vi "AIS Shielding Box Management.vi"() -> ()   [LabVIEW 2020]
uses:
  Commun VI/TypeDef/Commande Popup autotest/Commande element autotest.ctl
  01 - Structure de base/Fonction/Shielding Box/Action.ctl
  01 - Structure de base/Commande special/Exit.ctl
  01 - Structure de base/IHM/Variable globale.vi
panel:
  out "Element autotest":T1
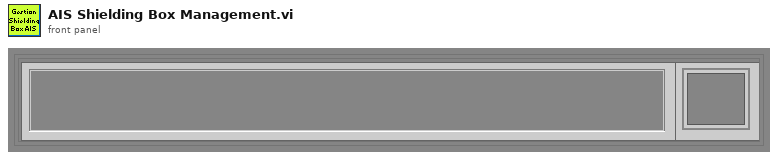
[diagram p1: front panel]
types:
  T1 = typedef "Commande element autotest.ctl" = cluster{"Instrument":string, "Etat":cluster{"Menu déroulant":u16}}
  T2 = typedef "Action.ctl" = enum16{"Open Shielding", "Close Shielding", "Read Status", "Stop Wait Start", "Wait Start", "Wait Close", "Wait Open", "Quit"}
  T3 = typedef "File et notification.ctl" = cluster{"Arret Appli":refnum<notifier>, "Erreur Acqui":refnum<notifier>, "File Event Sequenceur":refnum<queue>, "Liste test à faire":refnum<queue>, "File Event Historique":refnum<queue>, "Variable Global":refnum<notifier>, "Variable stocke retour Etat":refnum<notifier>, "Retour Validation OP":refnum<queue>, "Demande Validation OP":refnum<queue>, "Retour Autotest":refnum<notifier>, "Demande Autotest":refnum<queue>, "Adr Mac Produit":refnum<notifier>, "Autorise commande":refnum<notifier>, "Event Init BLE":refnum<notifier>, "Action Lecture RS":refnum<queue>, "Key produit":refnum<notifier>, "Retour Saisie OP":refnum<queue>, "Demande Saisie OP":refnum<queue>, "Etat flashage":refnum<notifier>, "Code Operateur":refnum<notifier>, "Resultat test Global":refnum<notifier>, "Stop Test":refnum<notifier>, "Init IHM Autotest":refnum<notifier>, "Version test bench":refnum<notifier>, "SN Product":refnum<notifier>, "En erreur":refnum<notifier>, "Affiche Result":refnum<queue>, "S/N PWR":refnum<notifier>, "AppEUI":refnum<notifier>, "Action Lecture Temp":refnum<queue>, "Temp":refnum<notifier>, "AppKey":refnum<notifier>, "OF":refnum<notifier>, "File Commande Shielding":refnum<queue>, "Return Status":refnum<notifier>, "ID Product":refnum<notifier>, "Version FW":refnum<notifier>, "Version HW":refnum<notifier>, "Adresse IHM":refnum<notifier>, "RTC":refnum<notifier>, "S/N Ant":refnum<notifier>, "SN Encode":refnum<notifier>, "Key Product":refnum<notifier>}
  T4 = typedef "Commande Variable Global.ctl" = cluster{"Fichier":cluster{"Chemin Save Historique":path, "Fichier Appplication":string, "Fichier Test":string, "Fichier Langue":string, "Part Number":string, "Fichier Parametre":string, "Chemin Fichier Parametre":path, "Fichier Print":string, "Fichier BDD":string}, "Liaison Serie":cluster{"RS Alimentation":refnum<visa-resource-name>, "RS Multimetre":refnum<k15>, "RS Carte":refnum<visa-resource-name>, "RS Dongle WIFI":refnum<visa-resource-name>, "RS Dongle BLE":refnum<visa-resource-name>, "RSA306":refnum<visa-resource-name>, "RS Printer PCBA":refnum<visa-resource-name>, "RS Golden Sample":refnum<visa-resource-name>, "RS Printer Ass":refnum<visa-resource-name>, "RS Printer Pack":refnum<visa-resource-name>, "RS Sonde Temp":refnum<visa-resource-name>, "RS Multimetre Bis":refnum<k15>, "RS FEASA LED":refnum<visa-resource-name>}, "Liaison DIO":cluster{"Jlink":cluster{"Line":tag, "Nom Voie":string, "Nom device in INI":string}[], "ICD":cluster{"Line":tag, "Nom Voie":string, "Nom device in INI":string}[], "UART":cluster{"Line":tag, "Nom Voie":string, "Nom device in INI":string}[], "Multi1":cluster{"Line":tag, "Nom Voie":string, "Nom device in INI":string}[], "Multi2":cluster{"Line":tag, "Nom Voie":string, "Nom device in INI":string}[], "Multi3":cluster{"Line":tag, "Nom Voie":string, "Nom device in INI":string}[], "DO1":cluster{"Line":tag, "Nom Voie":string, "Nom device in INI":string}[], "DO2":cluster{"Line":tag, "Nom Voie":string, "Nom device in INI":string}[], "DO3":cluster{"Line":tag, "Nom Voie":string, "Nom device in INI":string}[], "AlimProduct":cluster{"Line":tag, "Nom Voie":string, "Nom device in INI":string}[], "SW2":cluster{"Line":tag, "Nom Voie":string, "Nom device in INI":string}[], "SW1":cluster{"Line":tag, "Nom Voie":string, "Nom device in INI":string}[], "Multi220V_CPT":cluster{"Line":tag, "Nom Voie":string, "Nom device in INI":string}[]}, "Variable Programme":T5, "Information Entete":cluster{"Opérateur":string, "Ordre de fabrication":string, "Numéro de lot":string, "Commentaire":string}, "Nom de périphérique DAQmx":tag, "Parameter RF":cluster{"Frequency CW":string, "FrequencyRX":string, "TimeOutRX":string}, "Divers":cluster{"DUT Hub":u32}, "Analogique":cluster{"AI1":cluster{"Voie":tag, "Nom Voie":string, "Nom device in INI":string}[], "Ai2":cluster{"Voie":tag, "Nom Voie":string, "Nom device in INI":string}[], "AI3":cluster{"Voie":tag, "Nom Voie":string, "Nom device in INI":string}[], "AI4":cluster{"Voie":tag, "Nom Voie":string, "Nom device in INI":string}[], "AI5":cluster{"Voie":tag, "Nom Voie":string, "Nom device in INI":string}[], "AI6":cluster{"Voie":tag, "Nom Voie":string, "Nom device in INI":string}[], "AI7":cluster{"Voie":tag, "Nom Voie":string, "Nom device in INI":string}[], "AI8":cluster{"Voie":tag, "Nom Voie":string, "Nom device in INI":string}[], "AO1":cluster{"Voie":tag, "Nom Voie":string, "Nom device in INI":string}[], "AO2":cluster{"Voie":tag, "Nom Voie":string, "Nom device in INI":string}[]}, "Parametre BLE":T8, "Shielding Box":cluster{"Comm":refnum<visa-resource-name>, "Used":bool}, "Challenge Bit":u8[]}
  T5 = typedef "Commande Variables Programme.ctl" = cluster{"Cigarette en cours":i32, "Tableau Resultat test":T6, "Test en cours":i32, "Type test":string, "Type Carte":T7, "Test Select":cluster{"Booléen 4":bool}[]}
  T6 = typedef "Commande tableau Resultat.ctl" = cluster{"Resultat produit":cluster{"Nom test":string, "Result test":bool[], "Nom pointe de test":string[], "Valeur test":string[], "Temps Etape":dbl, "Numero Etape":string[]}[]}[]
  T7 = typedef "Commande Selection produit en cours.ctl" = enum16{"None", "PCBA", "Assembled"}
  T8 = typedef "Comande Variable Globale BLE.ctl" = cluster{"Devices Connect":string[][], "Connection Status":T9, "Handle table":string[][], "Service":string, "characteristic Read":string, "characteristic Write":string, "Port BLE":refnum<visa-resource-name>, "Nb Packet Light":u8}
  T9 = typedef "connection_status_bundle.ctl" = cluster{"MAC Address":string, "cnx handle":u8, "cnx flags":u8, "Address Type":T10, "Connection Interval (ms)":u16, "Timeout(ms)":u16, "Latency":u16, "bonding handle":u8}
  T10 = typedef "address_type.ctl" = u8
  T11 = typedef "Exit.ctl" = bool
  T12 = enum32{"Invalid", "Standard", "Closed", "Hidden", "Minimized", "Maximized"}
  T13 = typedef "Adresse IHM.ctl" = cluster{"TabGestionScénario":refnum<vi>, "MAJ TabTest":refnum<vi>, "MAJ IHM":refnum<vi>, "BpStop":refnum<vi>, "Autotest OK":refnum<vi>, "BpContinue":refnum<vi>, "BpStart":refnum<vi>, "Action en chinois":refnum<vi>, "Bouton vide":refnum<vi>, "StatusPCB":refnum<vi>, "StatusAssembled":refnum<vi>, "Bouton Exit":refnum<vi>, "Action En cours":refnum<vi>}
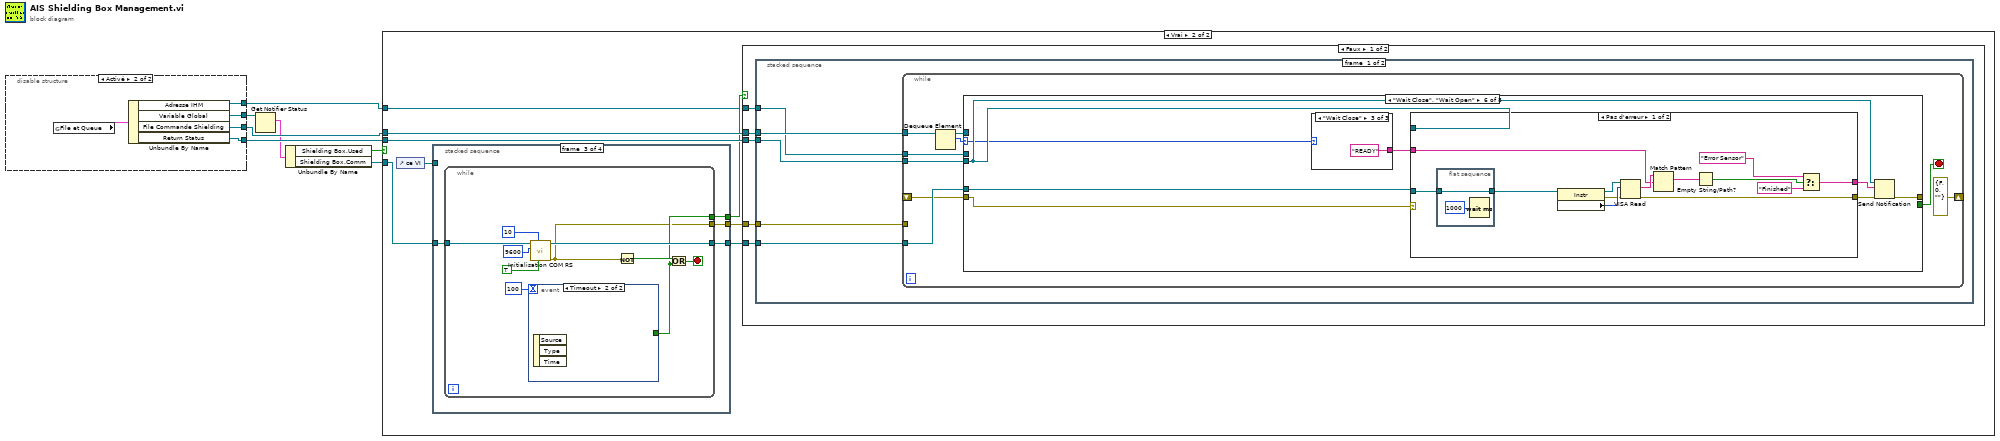
[diagram p0: block diagram]
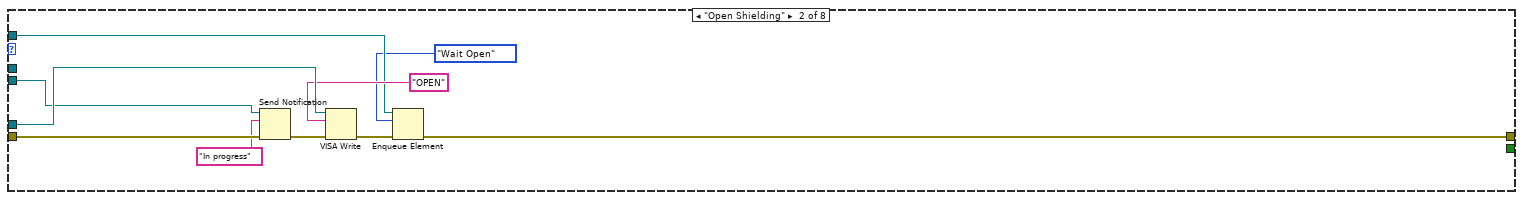
[diagram p4: hidden frame]
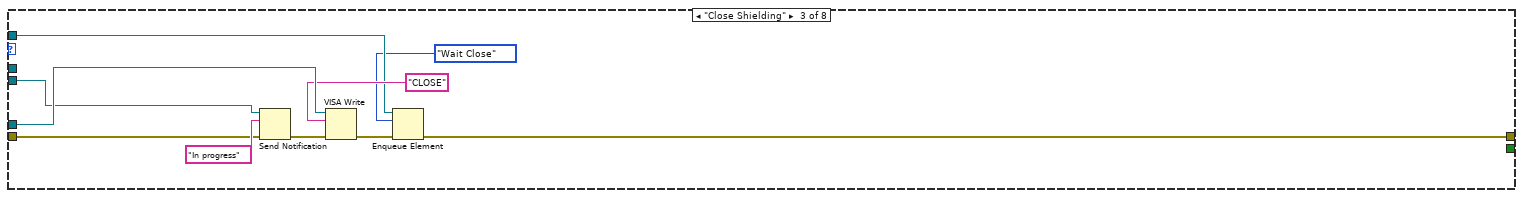
[diagram p5: hidden frame]
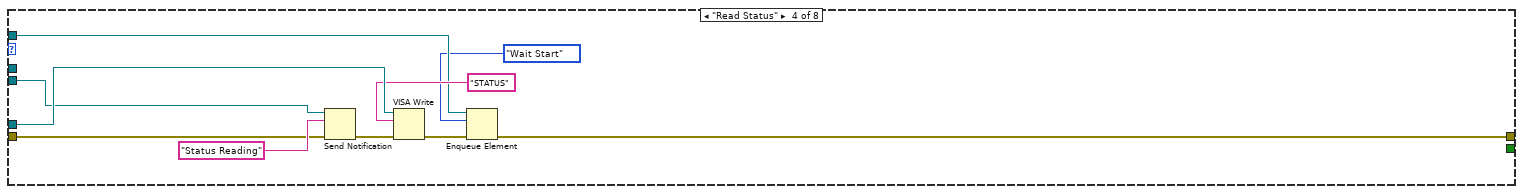
[diagram p6: hidden frame]
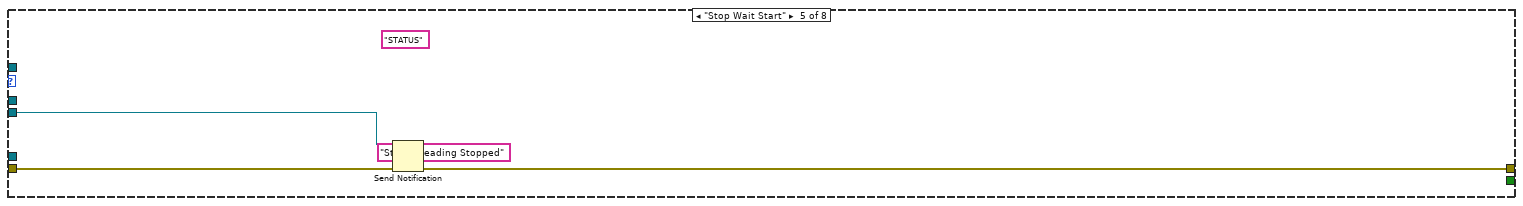
[diagram p7: hidden frame]
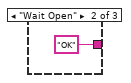
[diagram p9: hidden frame]
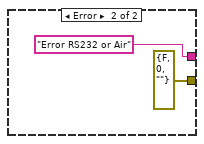
[diagram p10: hidden frame]
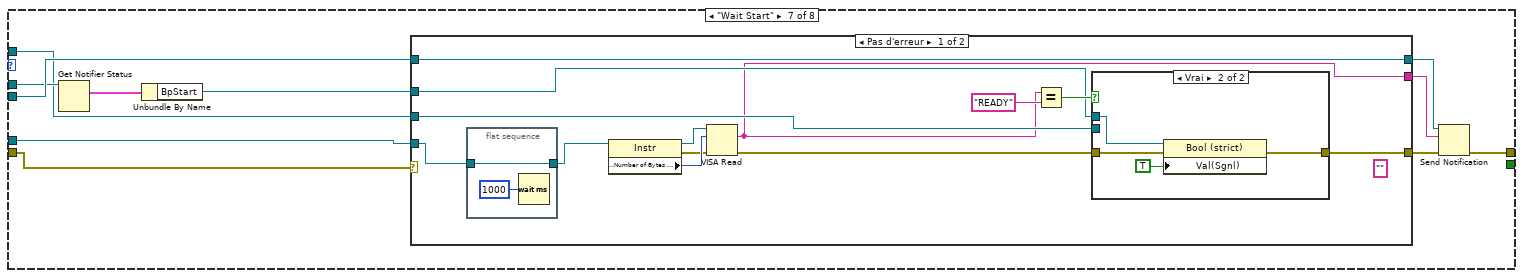
[diagram p11: hidden frame]
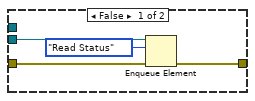
[diagram p12: hidden frame]
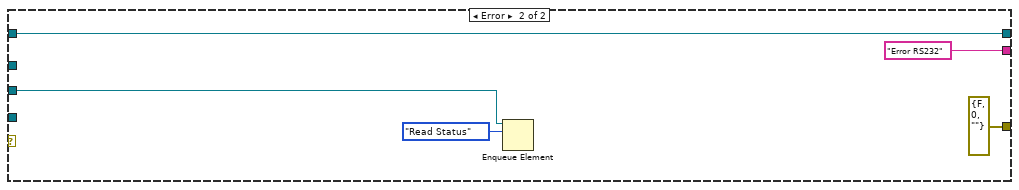
[diagram p13: hidden frame]
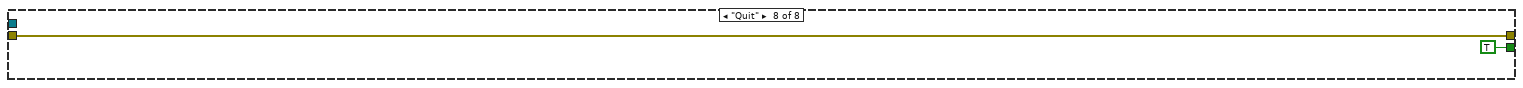
[diagram p14: hidden frame]
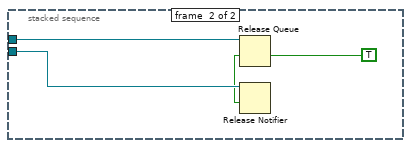
[diagram p15: hidden frame]
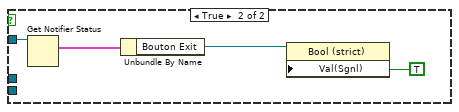
[diagram p16: hidden frame]
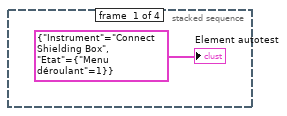
[diagram p17: hidden frame]
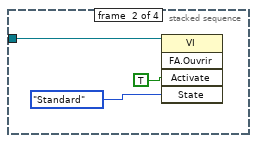
[diagram p18: hidden frame]
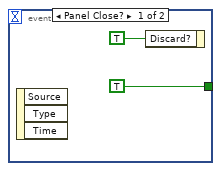
[diagram p19: hidden frame]
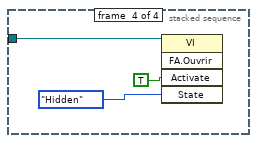
[diagram p20: hidden frame]
diagram:
  n1 = disable-structure shown="Activé" {
    disable-tunnel: [w12 w17] -> w7
    disable-tunnel: [w9 w16] -> w6
    disable-tunnel: [_ w15] -> w5
    disable-tunnel: [_ w14] -> w1
    frame Disabled {
      n2 = Obtain Queue(name (unnamed)="File Commande Shielding" ("nom (aucun)"), element data type=Action."Wait Start") -> (queue out=w12:refnum<queue>)  [unwired: 3 in, 2 out]
      n3 = Obtain Notifier(name (unnamed)="Return Status" ("nom (aucun)"), notification data type="") -> (notifier out=w9:refnum<notifier>)  [unwired: 2 in, 2 out]
    }
    frame Enabled {
      n4 = global read "Variable globale.vi" "File et Queue"() -> (w18:T3)
      n5 = Unbundle By Name(w18) -> ("Adresse IHM"=w14:refnum<notifier>, "Variable Global"=w15:refnum<notifier>, "File Commande Shielding"=w17:refnum<queue>, "Return Status"=w16:refnum<notifier>)
    }
  }
  n6 = Get Notifier Status(notifier=w5) -> (current notification=w3:T4)  [unwired: 1 in, 4 out]
  n7 = Unbundle By Name(w3) -> ("Shielding Box.Used"=w2:bool, "Shielding Box.Comm"=w4:refnum<visa-resource-name>)
  n8 = case shown="Vrai" w2 {
    tunnel: w7 -> [_ w26]
    tunnel: w6 -> [_ w25]
    tunnel: w1 -> [_ w20]
    tunnel: w4 -> [_ w19]
    frame False {
    }
    frame True {
      n9 = control-ref of="ce VI"() -> (w24:refnum<vi>)
      n10 = stacked-sequence {
        tunnel: w24 -> [_ w157 _ w176]
        tunnel: [_ _ w163 _] -> w23
        tunnel: [_ _ w162 _] -> w22
        tunnel: [_ _ w161 _] -> w21
        tunnel: w19 -> [_ _ w160 _]
        frame #0 {
          "Element autotest" <- T1 {"Instrument"="Connect Shielding Box", "Etat"={"Menu déroulant"=1}} ("Element autotest")
        }
        frame #1 {
          n11 = invoke class="VI" method="FA.Ouvrir"(reference=w157, "Activate"=TRUE ("Activer ?"), "State"=T12."Standard" ("État")) -> ()  [unwired: 2 in, 5 out]
        }
        frame #2 {
          n12 = while {
            tunnel: [w164] -> w163
            tunnel: [w170] -> w162
            tunnel: [w167] -> w161
            tunnel: w160 -> [w165]
            stop <- w169 stop-if-true
            n13 = event shown="[1] Timeout" {
              selector: _ -> [_ _]
              dyn-events: _ -> [_ _]
              timeout: 100 -> [_ _]
              tunnel: [TRUE _] -> w167
              event Panel Close? {
                n14 = event-data() -> ()  [unwired: 1 in, 3 out]
                n15 = event-data("Discard?"=TRUE ("Rejeter ?")) -> ()  [unwired: 1 in, 1 out]
              }
              event Timeout {
                n16 = event-data() -> ()  [unwired: 1 in, 3 out]
              }
            }
            n17 = call "Initialisation COM RS.vi"("Enable Termination\nChar (T)"=TRUE ("Enable Termination\nChar (T)"), "termination char\n(0xA = '\\n' = LF)"=u8 10 ("termination char\n(0xA = '\\n' = LF)"), "baud rate (9600)"=9600, "Refnum VISA en entrée"=w165) -> ("sortie d'erreur"=w164:errorcluster, "Nom de ressource VISA en sortie"=w170:refnum<visa-resource-name>)  [unwired: 6 in]
            n18 = Not(x=w164) -> (.not. x?=w168:bool)
            n19 = Or(x=w168, y=w167) -> (x .or. y?=w169:bool)
          }
        }
        frame #3 {
          n20 = invoke class="VI" method="FA.Ouvrir"(reference=w176, "Activate"=TRUE ("Activer ?"), "State"=T12."Hidden" ("État")) -> ()  [unwired: 2 in, 5 out]
        }
      }
      n21 = case shown="Faux" w21 {
        tunnel: w26 -> [w31 _]
        tunnel: w25 -> [w30 _]
        tunnel: w23 -> [w29 _]
        tunnel: w22 -> [w28 _]
        tunnel: w20 -> [w27 w155]
        frame False {
          n22 = stacked-sequence {
            tunnel: w28 -> [w36 _]
            tunnel: w31 -> [w35 w151]
            tunnel: w29 -> [w34 _]
            tunnel: w30 -> [w33 w150]
            tunnel: w27 -> [w32 _]
            frame #0 {
              n23 = while {
                tunnel: w36 -> [w43]
                tunnel: w35 -> [w45]
                shift-right: [errorcluster {"status"=FALSE, "code"=0, "source"=""} ("error out")] -> _
                shift-left: _ -> [w42]
                tunnel: w34 -> [_]
                tunnel: w33 -> [w39]
                tunnel: w32 -> [w37]
                stop <- w40 stop-if-true
                n24 = Dequeue Element(queue=w45) -> (queue out=w41:refnum<queue>, element=w44:T2)  [unwired: 2 in, 2 out]
                n25 = case shown="\"Wait Close\", \"Wait Open\"" w44 {
                  selector: w44 -> [_ _ _ _ _ w86 _ _]
                  tunnel: w43 -> [_ w56 w66 w76 _ w88 w118 _]
                  tunnel: w42 -> [w46 w54 w58 w68 w78 w81 w108 w148]
                  tunnel: [w46 w52 w63 w73 w77 w82 w114 w148] -> _
                  tunnel: w41 -> [_ w51 w62 w72 _ _ w110 _]
                  tunnel: [_ _ _ _ _ _ _ TRUE] -> w40
                  tunnel: w39 -> [_ w48 w59 w69 w79 w87 w117 _]
                  tunnel: w37 -> [_ _ _ _ _ _ w115 _]
                  frame Default {
                  }
                  frame "Open Shielding" {
                    n26 = Send Notification(notification="In progress", notifier=w48, error in (no error)=w54) -> (error out=w49:errorcluster)  [unwired: 1 out]
                    n27 = VISA Write(VISA resource name=w56, write buffer="OPEN" ("buffer d'écriture"), error in (no error)=w49) -> (error out=w53:errorcluster)  [unwired: 2 out]
                    n28 = Enqueue Element(queue=w51, element=Action."Wait Open" ("élément"), error in (no error)=w53) -> (error out=w52:errorcluster)  [unwired: 1 in, 2 out]
                  }
                  frame "Close Shielding" {
                    n29 = Send Notification(notification="In progress", notifier=w59, error in (no error)=w58) -> (error out=w57:errorcluster)  [unwired: 1 out]
                    n30 = VISA Write(VISA resource name=w66, write buffer="CLOSE" ("buffer d'écriture"), error in (no error)=w57) -> (error out=w64:errorcluster)  [unwired: 2 out]
                    n31 = Enqueue Element(queue=w62, element=Action."Wait Close" ("élément"), error in (no error)=w64) -> (error out=w63:errorcluster)  [unwired: 1 in, 2 out]
                  }
                  frame "Read Status" {
                    n32 = Send Notification(notification="Status Reading", notifier=w69, error in (no error)=w68) -> (error out=w67:errorcluster)  [unwired: 1 out]
                    n33 = VISA Write(VISA resource name=w76, write buffer="STATUS" ("buffer d'écriture"), error in (no error)=w67) -> (error out=w74:errorcluster)  [unwired: 2 out]
                    n34 = Enqueue Element(queue=w72, element=Action."Wait Start" ("élément"), error in (no error)=w74) -> (error out=w73:errorcluster)  [unwired: 1 in, 2 out]
                  }
                  frame "Stop Wait Start" {
                    (unwired) "STATUS" ("buffer d'écriture")
                    n35 = Send Notification(notification="Status Reading Stopped", notifier=w79, error in (no error)=w78) -> (error out=w77:errorcluster)  [unwired: 1 out]
                  }
                  frame "Wait Close", "Wait Open" {
                    n36 = case shown="\"Wait Close\"" w86 {
                      tunnel: [_ "OK" ("expression régulière") "READY" ("expression régulière")] -> w85
                      frame Default {
                      }
                      frame "Wait Open" {
                      }
                      frame "Wait Close" {
                      }
                    }
                    n37 = case shown="Pas d'erreur" w81 {
                      tunnel: w88 -> [w92 _]
                      tunnel: w87 -> [_ _]
                      tunnel: w85 -> [w95 _]
                      tunnel: [w94 "Error RS232 or Air" ("cas faux")] -> w84
                      tunnel: [w93 errorcluster {"status"=FALSE, "code"=0, "source"=""} ("error out")] -> w83
                      frame No Error {
                        n38 = flat-sequence {
                          tunnel: w92 -> [w105]
                          tunnel: [w105] -> w91
                          frame #0 {
                            n39 = Wait (ms)(milliseconds to wait=u32 1000) -> ()  [unwired: 1 out]
                          }
                        }
                        n40 = property class="Instr"(reference=w91) -> (reference out=w103:refnum<visa-resource-name>, error out=w100:errorcluster, "Serial Settings:Number of Bytes at Serial Port"=w102:u32)  [unwired: 1 in]
                        n41 = VISA Read(VISA resource name=w103, byte count=w102, error in (no error)=w100) -> (read buffer=w99:string, error out=w93:errorcluster)  [unwired: 2 out]
                        n42 = Match Pattern(string=w99, regular expression=w95) -> (match substring=w101:string)  [unwired: 1 in, 3 out]
                        n43 = Empty String/Path?(string/path=w101) -> (empty?=w96:bool)
                        n44 = Select(t="Error Sensor" ("notification"), s=w96, f="Finished" ("cas faux")) -> (s? t:f=w94:string)
                      }
                      frame Error {
                      }
                    }
                    n45 = Send Notification(notification=w84, notifier=w87, error in (no error)=w83) -> (error out=w82:errorcluster)  [unwired: 1 out]
                  }
                  frame "Wait Start" {
                    n46 = Get Notifier Status(notifier=w115) -> (current notification=w116:T13)  [unwired: 1 in, 4 out]
                    n47 = Unbundle By Name(w116) -> ("BpStart"=w111:refnum<vi>)
                    n48 = case shown="Pas d'erreur" w108 {
                      tunnel: w118 -> [w120 _]
                      tunnel: w117 -> [w127 w144]
                      tunnel: [w121 "Error RS232" ("cas faux")] -> w112
                      tunnel: [w122 errorcluster {"status"=FALSE, "code"=0, "source"=""} ("error out")] -> w109
                      tunnel: [w127 w144] -> w113
                      tunnel: w111 -> [w125 _]
                      tunnel: w110 -> [w123 w142]
                      frame No Error {
                        (unwired) "" ("sous-chaîne")
                        n49 = flat-sequence {
                          tunnel: w120 -> [w133]
                          tunnel: [w133] -> w119
                          frame #0 {
                            n50 = Wait (ms)(milliseconds to wait=u32 1000) -> ()  [unwired: 1 out]
                          }
                        }
                        n51 = property class="Instr"(reference=w119) -> (reference out=w131:refnum<visa-resource-name>, error out=w129:errorcluster, "Serial Settings:Number of Bytes at Serial Port"=w130:u32)  [unwired: 1 in]
                        n52 = VISA Read(VISA resource name=w131, byte count=w130, error in (no error)=w129) -> (read buffer=w121:string, error out=w124:errorcluster)  [unwired: 2 out]
                        n53 = Equal?(x=w121, y="READY") -> (x = y?=w126:bool)
                        n54 = case shown="Vrai" w126 {
                          tunnel: w125 -> [_ w141]
                          tunnel: w124 -> [w137 w139]
                          tunnel: [w136 w138] -> w122
                          tunnel: w123 -> [w135 _]
                          frame False {
                            n55 = Enqueue Element(queue=w135, element=Action."Read Status" ("élément"), error in (no error)=w137) -> (error out=w136:errorcluster)  [unwired: 1 in, 2 out]
                          }
                          frame True {
                            n56 = property class="Bool (strict)"(reference=w141, error in=w139, "Val(Sgnl)"=T11 TRUE ("Valeur (Signalisation)")) -> (error out=w138:errorcluster)  [unwired: 1 out]
                          }
                        }
                      }
                      frame Error {
                        n57 = Enqueue Element(queue=w142, element=Action."Read Status" ("élément")) -> ()  [unwired: 2 in, 3 out]
                      }
                    }
                    n58 = Send Notification(notification=w112, notifier=w113, error in (no error)=w109) -> (error out=w114:errorcluster)  [unwired: 1 out]
                  }
                  frame "Quit" {
                  }
                }
              }
            }
            frame #1 {
              w149 = TRUE ("forcer la destruction ? (F)")
              n59 = Release Queue(queue=w151, force destroy? (F)=w149) -> ()  [unwired: 1 in, 3 out]
              n60 = Release Notifier(notifier=w150, force destroy? (F)=w149) -> ()  [unwired: 1 in, 3 out]
            }
          }
        }
        frame True {
          n61 = Get Notifier Status(notifier=w155) -> (current notification=w152:T13)  [unwired: 1 in, 4 out]
          n62 = Unbundle By Name(w152) -> ("Bouton Exit"=w154:refnum<vi>)
          n63 = property class="Bool (strict)"(reference=w154, "Val(Sgnl)"=T11 TRUE ("Valeur (Signalisation)")) -> ()  [unwired: 1 in, 2 out]
        }
      }
    }
  }
